vi "digital write.vi"(8 "error in (no error)":errorcluster, 9 "On/Off":bool, 10 "Line":string, 11 "USB-6000 in":refnum<class "USB-6000.lvclass">) -> (0 "error out":errorcluster, 3 "USB-6000 out":refnum<class "USB-6000.lvclass">)   [LabVIEW 2025, in "USB IO.lvlib" / "USB-6000.lvclass"]
uses:
  USB-6000.lvclass
  USB-6000.lvclass/USB-6000.ctl
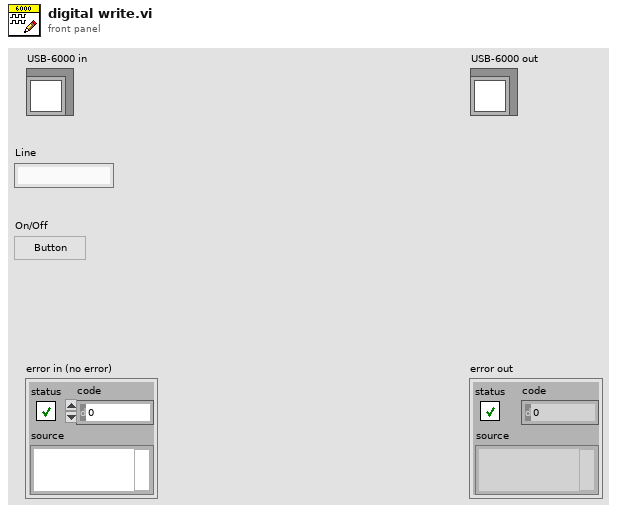
[diagram p1: front panel]
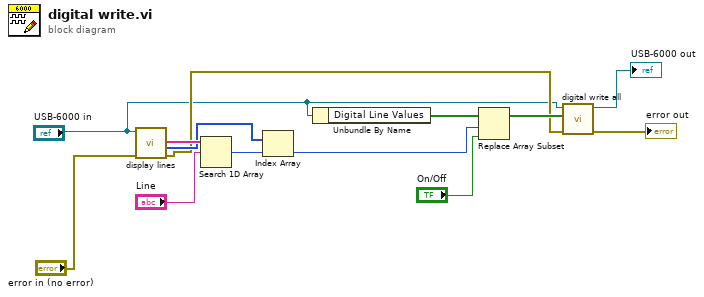
[diagram p0: block diagram]
diagram:
  n1 = call-dynamic "display lines.vi"("error in (no error)"="error in (no error)", "USB-6000 in"="USB-6000 in") -> ("error out"=w2:errorcluster, "Values"=w9:i32[], "Lines"=w11:string[])  [unwired: 6 in, 1 out]
  n2 = Search 1D Array(1D array=w11, element="Line") -> (index of element=w8:i32)  [unwired: 1 in]
  n3 = Index Array(array=w9, index=w8) -> (element=w6:i32)
  n4 = Unbundle By Name("USB-6000 in") -> ("Digital Line Values"=w7:bool[])
  n5 = Replace Array Subset(array=w7, new element="On/Off", index=w6) -> (w4:bool[])
  n6 = call "digital write all.vi"("error in (no error)"=w2, "data"=w4, "USB-6000 in"="USB-6000 in") -> ("error out"=→"error out":errorcluster, "USB-6000 out"=→"USB-6000 out":refnum<class "USB-6000.lvclass">)  [unwired: 7 in]
